vi "Initiate Updates.vi"(8 "error in (no error)":errorcluster, 11 "IController In":refnum<class "IController.lvclass">) -> (0 "error out":errorcluster, 3 "IController Out":refnum<class "IController.lvclass">)   [LabVIEW 2015, in "IController.lvlib" / "IController.lvclass"]
uses:
  IController.lvclass
  IViewable/IViewable/IViewable.lvclass/IViewable.ctl
  IViewManager/IViewManager/IViewManager.lvclass
  IViewable/IViewable/IViewable.lvclass
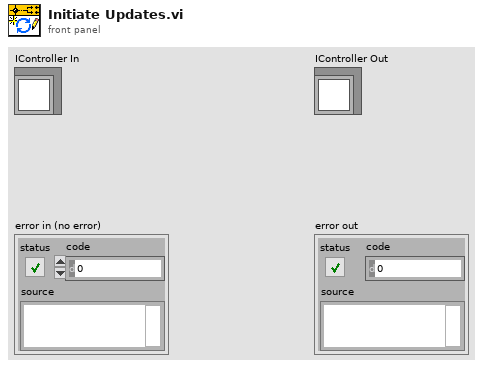
[diagram p1: front panel]
types:
  T1 = enum32{"Invalid", "Standard", "Closed", "Hidden", "Minimized", "Maximized"}
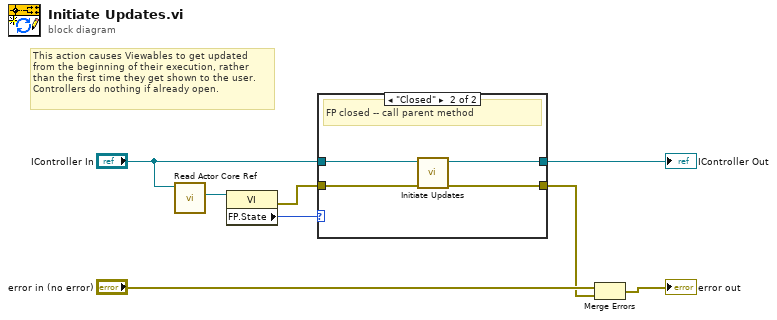
[diagram p0: block diagram]
diagram:
  # "This action causes Viewables to get updated\nfrom the beginning of their execution, rather\nthan the first time they get shown to the user.\nControllers do nothing if already open."
  n1 = call "Read Actor Core Ref.vi"("IViewable In"="IController In") -> ("Actor Core Ref"=w6:refnum<vi>)  [unwired: 8 in, 2 out]
  n2 = property class="VI"(reference=w6) -> (error out=w1:errorcluster, "FP.State"=w3:T1)  [unwired: 1 in, 1 out]
  n3 = case shown="\"Closed\"" w3 {
    tunnel: "IController In" -> [w10 w14]
    tunnel: [w10 w13] -> w4
    tunnel: [w9 w12] -> w2
    tunnel: w1 -> [w9 w11]
    frame Default {
      # "FP not closed -- do nothing"
    }
    frame "Closed" {
      # "FP closed -- call parent method"
      n4 = call-parent "Initiate Updates.vi"("error in (no error)"=w11, "IViewable In"=w14) -> ("error out"=w12:errorcluster, "IViewable Out"=w13:refnum<class "IController.lvclass">)  [unwired: 8 in]
    }
  }
  "IController Out" <- w4
  n5 = Merge Errors("error in (no error)", w2) -> (→"error out":errorcluster)
